vi "SVPO TDMS Write SGL Waveform (N Ch).vi"(0 "tdms file":refnum<k34>, 1 "write channel properties? (T)":bool=TRUE, 5 "group name in":string="Waveforms", 7 "channel names in":string[](array[string]), 9 "scaled signals [EU]":waveform(sgl)[](array[waveform])) -> (4 "tdms file out":refnum<k34>, 6 "group name out":string, 8 "channel names out":string[](array[string]))   [LabVIEW 2017]
doc: "Writes single-precision waveform or scaled array data to the specified .tdms file in a format specific to the polymorphic instance. Use this VI on embedded targets that have limited computational resources. Wire data to the <B>scaled signal [EU]</B> input to determine the polymorphic instance to use or manually select the instance."
uses:
  <vilib>/addons/_NISVFA/_Shared subVIs/Controls/LV Datatypes.ctl
  <vilib>/addons/_NISVFA/_Shared subVIs/Controls/NI Function Info.ctl
  <vilib>/addons/_NISVFA/_Shared subVIs/Controls/NI Function Type.ctl
  <vilib>/addons/_NISVFA/_Shared subVIs/Controls/NI Function SubType.ctl
  <vilib>/addons/_NISVFA/_Shared subVIs/Controls/svc_X-Axis Units.ctl
  <vilib>/addons/_NISVFA/_Shared subVIs/Controls/svc_Unit Info.ctl
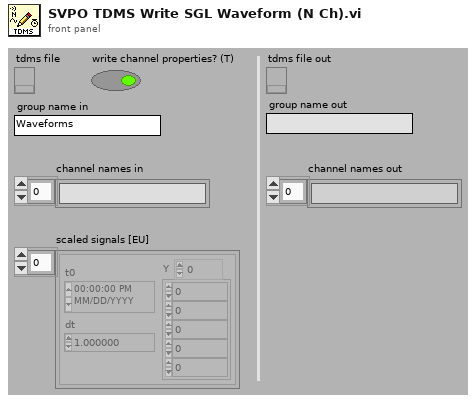
[diagram p1: front panel]
types:
  T1 = typedef "NI Function Info.ctl" = cluster{"function type":T2, "function subtype":T3, "X-dimension":T4}
  T2 = typedef "NI Function Type.ctl" = u16
  T3 = typedef "NI Function SubType.ctl" = u16
  T4 = typedef "svc_X-Axis Units.ctl" = u16
  T5 = typedef "LV Datatypes.ctl" = i32
  T6 = typedef "svc_Unit Info.ctl" = cluster{"X-axis label":string, "X-unit string":string, "Y-axis label":string, "Y-unit string":string}
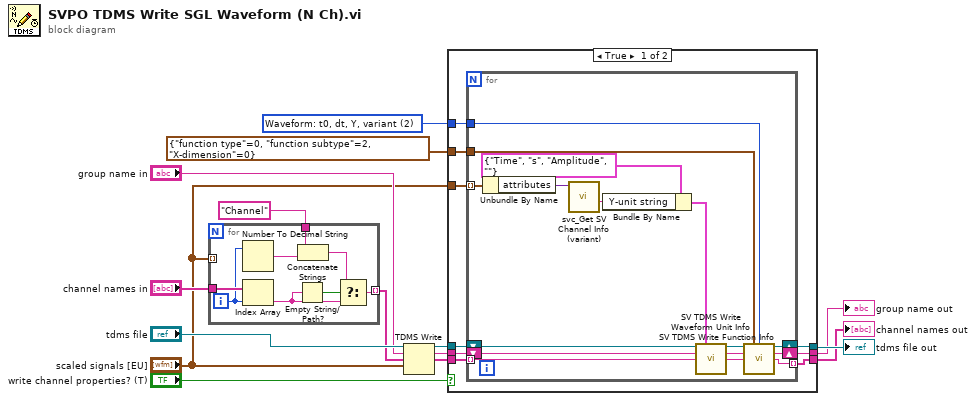
[diagram p0: block diagram]
diagram:
  w4 = T5 2 items=["String: abc"=-2, "Boolean: True or False"=-1, "Scalar: y"=0, "Array: Y"=1, "Waveform: t0, dt, Y, variant"=2, "Cluster: x0, dx, Y"=3, "Cluster: X, Y"=4, "Waterfall"=5, "Colormap"=6] ("LabVIEW datatype")
  n1 = for {
    tunnel: "channel names in" -> [w23]
    tunnel: [w22] -> w5 mode=indexing
    tunnel: "Channel" ("string") -> [w16]
    tunnel: "scaled signals [EU]" -> [_] mode=indexing
    i -> [w19]
    n2 = Number To Decimal String(number=w19) -> (decimal integer string=w18:string)  [unwired: 1 in]
    n3 = Index Array(array=w23, index=w19) -> (element=w20:string)
    n4 = Empty String/Path?(string/path=w20) -> (empty?=w21:bool)
    n5 = Concatenate Strings(w16, w18) -> (w17:string)
    n6 = Select(t=w17, s=w21, f=w20) -> (s? t:f=w22:string)
  }
  n7 = TDMS Write(0:"tdms file", 5:"group name in", 7:w5, 9:"scaled signals [EU]") -> (4:w11:refnum<k34>, 6:w9:string, 8:w8:string[])  [unwired: 2 in, 1 out]
  n8 = case shown="True" "write channel properties? (T)" {
    tunnel: [w32 w51] -> w15
    tunnel: w11 -> [w31 w51]
    tunnel: [w26 w50] -> w14
    tunnel: [w25 w49] -> w13
    tunnel: w9 -> [w30 w50]
    tunnel: w8 -> [w29 w49]
    tunnel: T1 {"function type"=0, "function subtype"=2, "X-dimension"=0} ("function info") -> [w28 _]
    tunnel: w4 -> [w27 _]
    tunnel: "scaled signals [EU]" -> [w24 _]
    frame True {
      n9 = for {
        shift-right: [w36] -> w32
        shift-left: w31 -> [w46]
        tunnel: w29 -> [w44] mode=indexing
        tunnel: w28 -> [w42]
        tunnel: w27 -> [w43]
        tunnel: [w37] -> w25 mode=indexing
        shift-right: [w38] -> w26
        shift-left: w30 -> [w45]
        tunnel: w24 -> [w48] mode=indexing
        n10 = Unbundle By Name(w48) -> ("attributes"=w47:variant)
        n11 = call <vilib>:"svc_Get SV Channel Info (variant).vi"("attributes"=w47) -> ("unit label"=w34:string)  [unwired: 5 in, 5 out]
        n12 = Bundle By Name(cluster=T6 {"X-axis label"="Time", "X-unit string"="s", "Y-axis label"="Amplitude", "Y-unit string"=""} ("unit info"), "Y-unit string"=w34) -> (w33:T6)
        n13 = call <vilib>:"SV TDMS Write Waveform Unit Info.vi"("tdms file"=w46, "unit info"=w33, "group name"=w45, "channel name"=w44) -> ("tdms file out"=w41:refnum<k34>, "group name out"=w40:string, "channel name out"=w39:string)  [unwired: 8 in, 1 out]
        n14 = call <vilib>:"SV TDMS Write Function Info.vi"("tdms file in"=w41, "function info"=w42, "LabVIEW datatype"=w43, "group name"=w40, "channel name"=w39) -> ("tdms file out"=w36:refnum<k34>, "group name out"=w38:string, "channel name out"=w37:string)  [unwired: 7 in, 1 out]
      }
    }
    frame False {
    }
  }
  "tdms file out" <- w15
  "channel names out" <- w13
  "group name out" <- w14
